vi "LABWAD.vi"() -> ()   [LabVIEW 2017]
uses:
  SubVIs/WAD_MainCluster.ctl
  SubVIs/TextureList.ctl
  SubVIs/PatchList.ctl
  SubVIs/Lumps.ctl
  Fire/Spread Fire.vi
  <vilib>/picture/picture.llb/Draw 8-Bit Pixmap.vi
  <userlib>/_OpenG.lib/array/array.llb/Filter 1D Array (String)__ogtk.vi
  <userlib>/_OpenG.lib/array/array.llb/Filter 1D Array with Scalar (String)__ogtk.vi
  <vilib>/regexp/Match Regular Expression.xnode
panel:
  out "2D Picture":picture
  in  "File Structure":string[](tree)
  out "Demonic Intensity Graph":i32[][](graph)
  # "Overview: Demonstrates how to read WAD files from original DOOM games.\nRequirements: LabVIEW Full Development System 2017 or compatible\nInstructions:\n1. Run this VI.\n2. Select a .wad file using the File > Open WAD File menu.\n3. Click on different items in the tree view to display them.\n4. Export the displayed image as PNG via drop-down menu on picture, or\n    select and export multiple items from the tree list via drop-down menu.\n5. Quit by using the File > Quit menu."
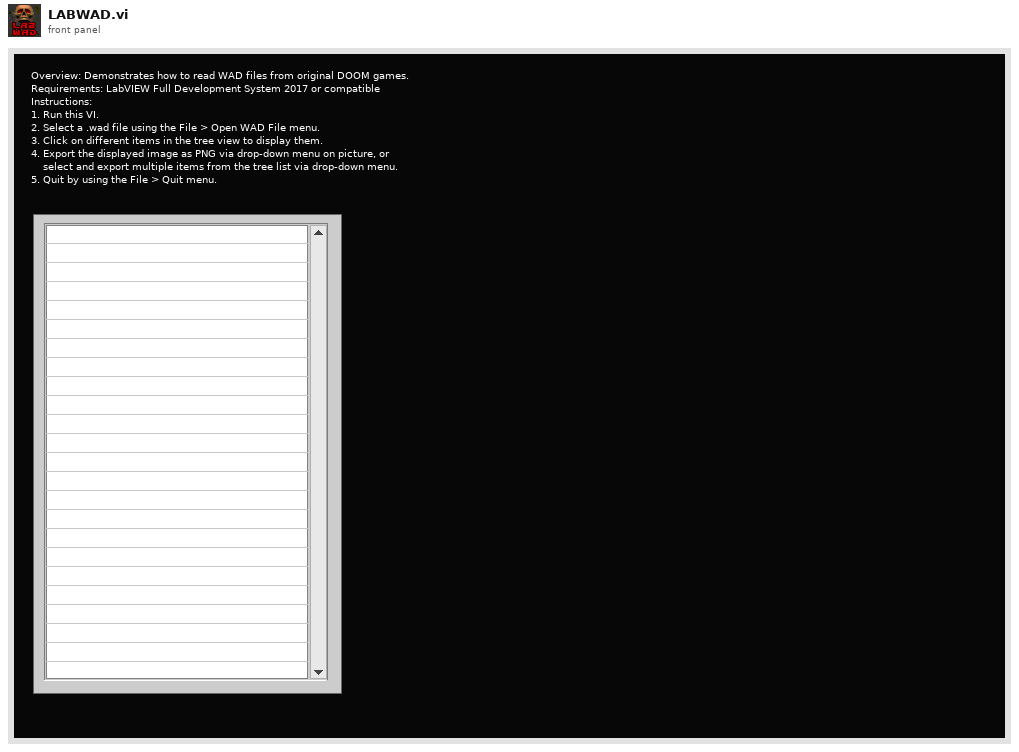
[diagram p1: front panel]
types:
  T1 = typedef "WAD_MainCluster.ctl" = cluster{"WAD file path":path, "WAD as U8 Array":u8[], "WAD Tree":refnum<vi>, "Palette":u32[], "TextureList":T2[], "PNAMES":string[], "Image Array":i16[][], "2D Picture":picture, "Lumps List":string[], "Lumps Array":T4[], "Textures Names":string[], "Image Mask":i16[][], "S_START Index":i32}
  T2 = typedef "TextureList.ctl" = cluster{"Name":string, "flags":u16, "masked":i16, "width":i16, "height":i16, "columndirectory":u32, "patchcount":i16, "PatchList":T3[]}
  T3 = typedef "PatchList.ctl" = cluster{"originx":i16, "originy":i16, "patch":i16}
  T4 = typedef "Lumps.ctl" = cluster{"offData":i32, "lenData":i32, "name":string}
  T5 = typedef "imagedata.ctl" = cluster{"image type":i32, "image depth":i32, "image":u8[], "mask":u8[], "colors":u32[], "Rectangle":cluster{"left":i16, "top":i16, "right":i16, "bottom":i16}}
  T6 = typedef "PatchHeader.ctl" = cluster{"Width":u16, "Height":u16, "XOffset":i16, "YOffset":i16}
  T7 = typedef "LVBoundsTypeDef.ctl" = cluster{"Width":u32, "Height":u32}
  T8 = cluster{"ItemTag":string, "Navigate Tree:Get Path":string[][]}
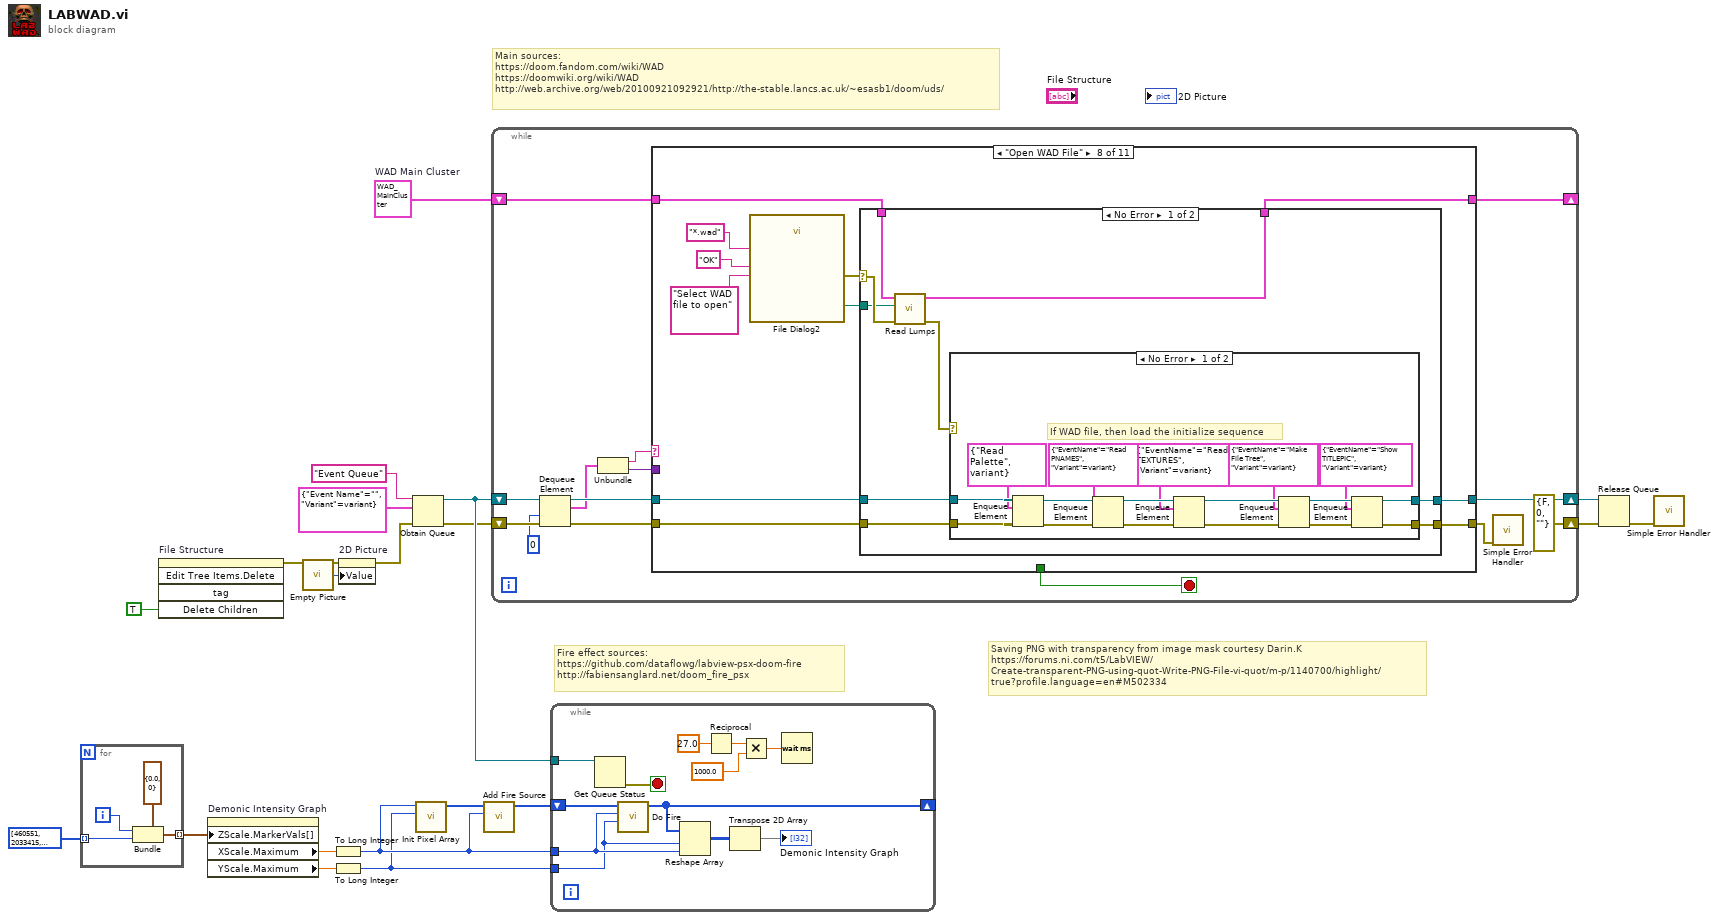
[diagram p0: block diagram]
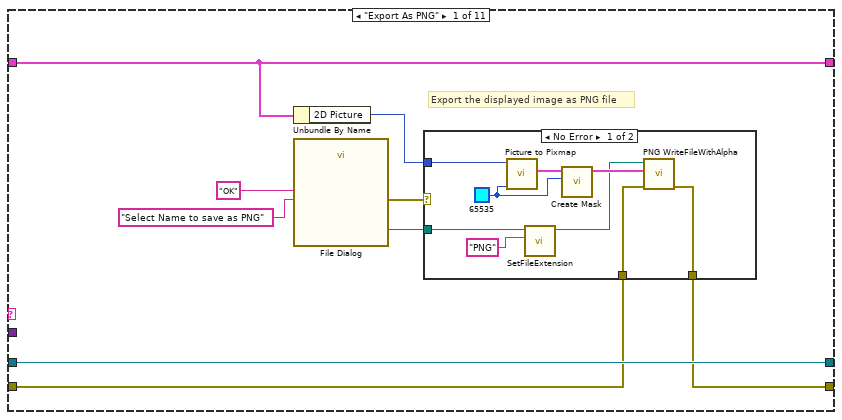
[diagram p2: hidden frame]
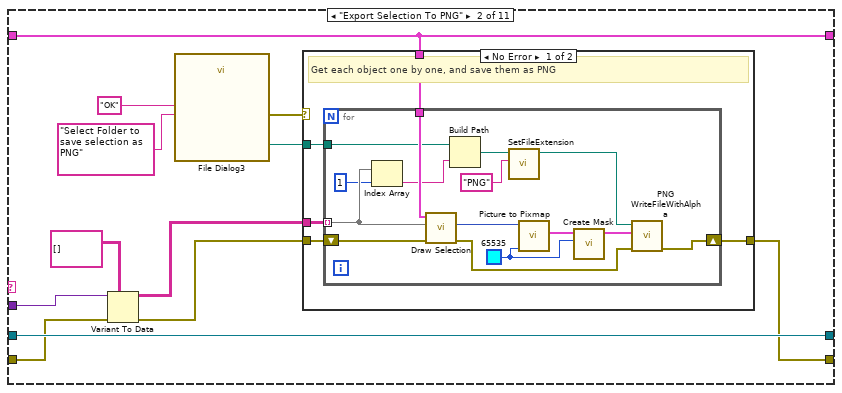
[diagram p4: hidden frame]
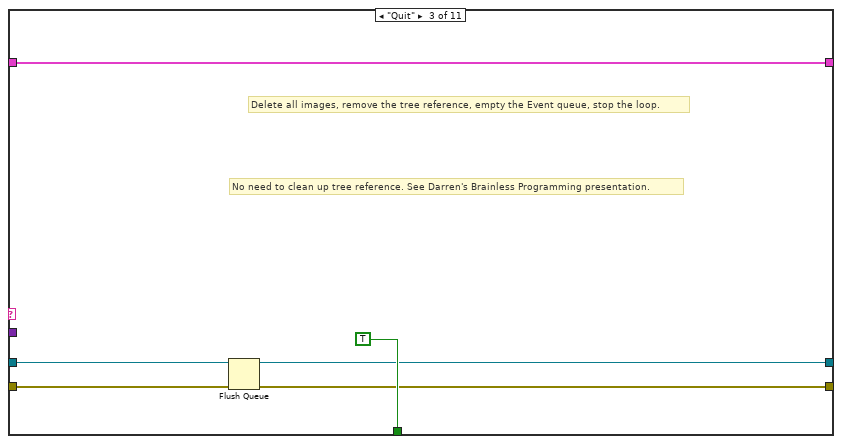
[diagram p6: hidden frame]
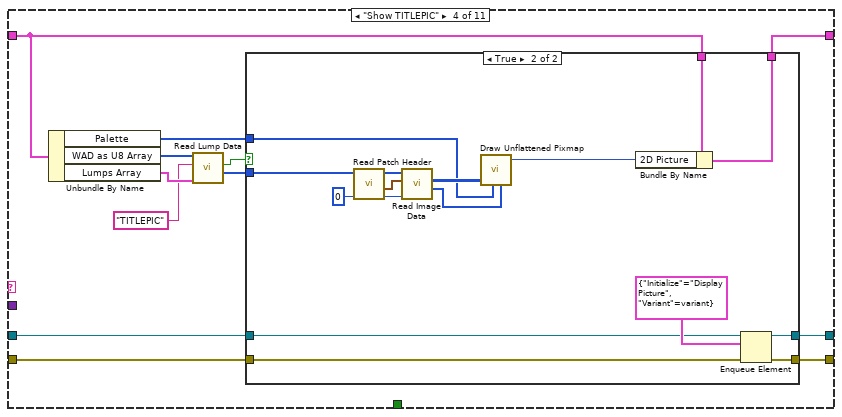
[diagram p7: hidden frame]
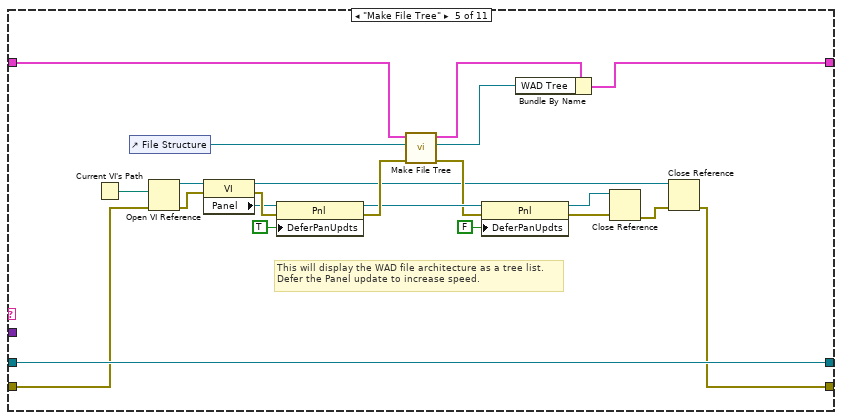
[diagram p9: hidden frame]
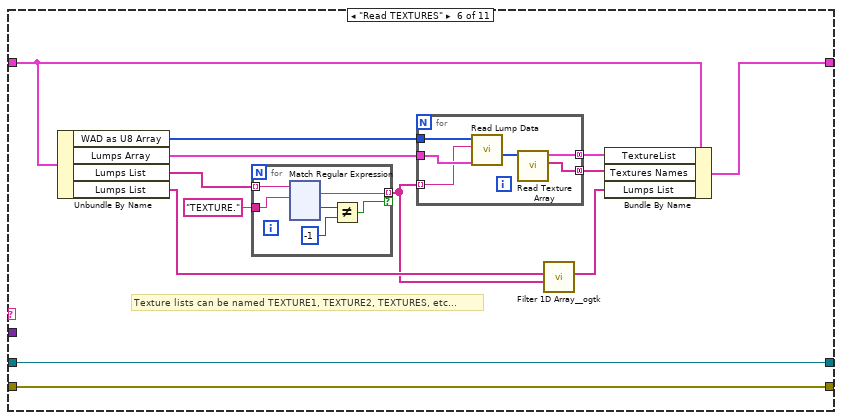
[diagram p10: hidden frame]
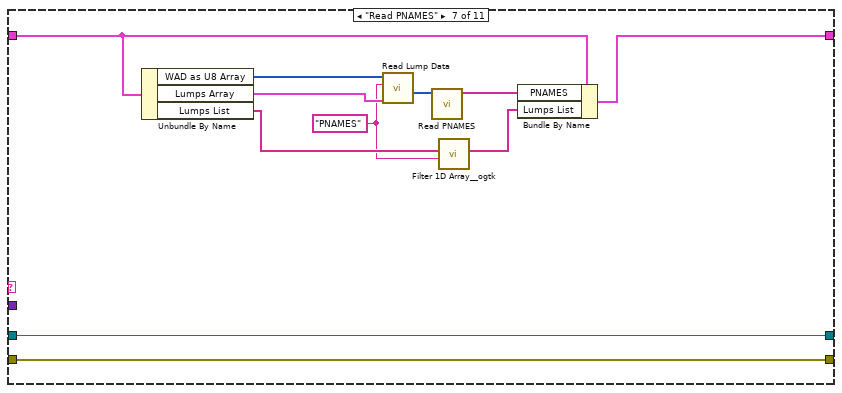
[diagram p11: hidden frame]
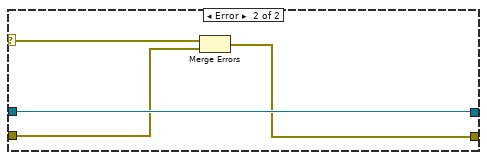
[diagram p12: hidden frame]
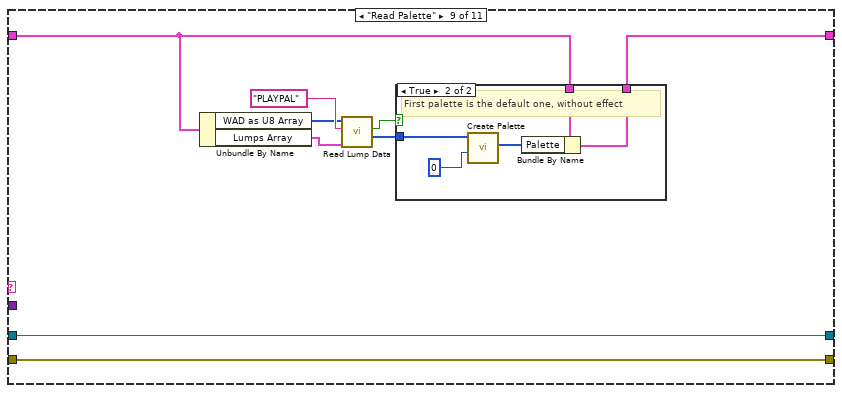
[diagram p14: hidden frame]
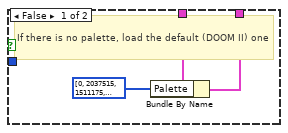
[diagram p15: hidden frame]
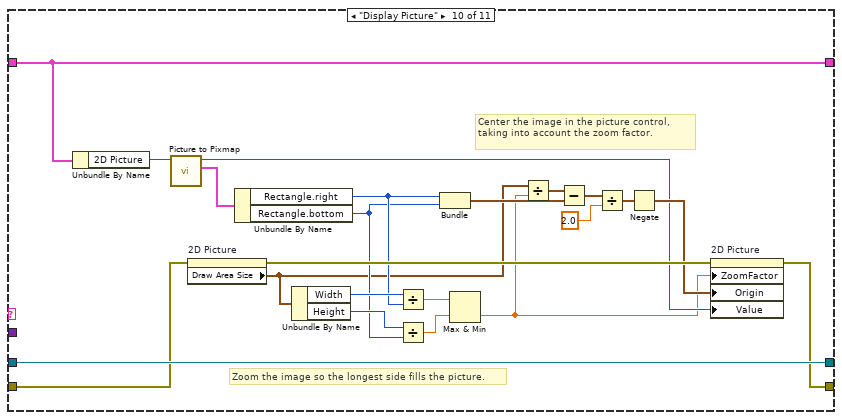
[diagram p16: hidden frame]
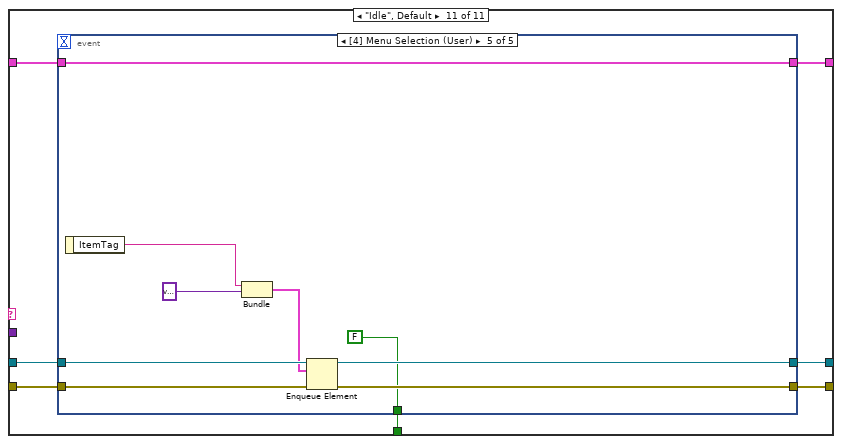
[diagram p17: hidden frame]
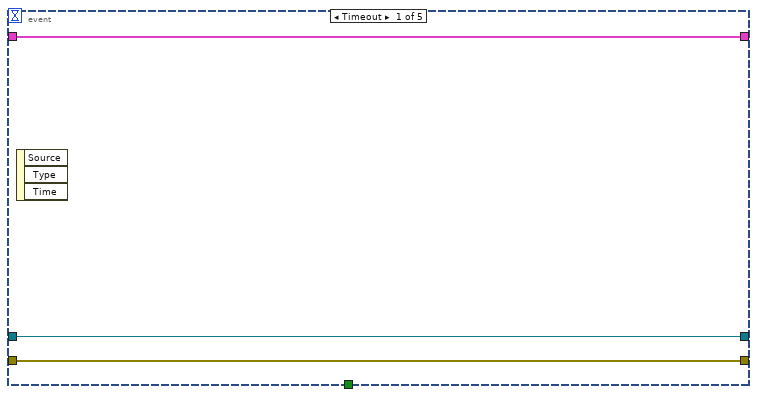
[diagram p18: hidden frame]
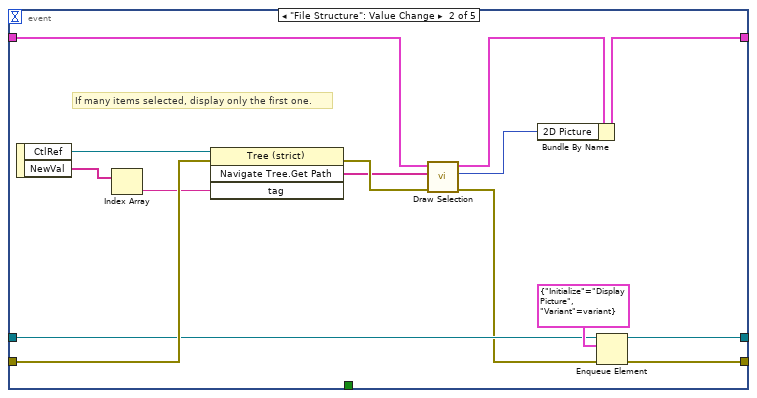
[diagram p19: hidden frame]
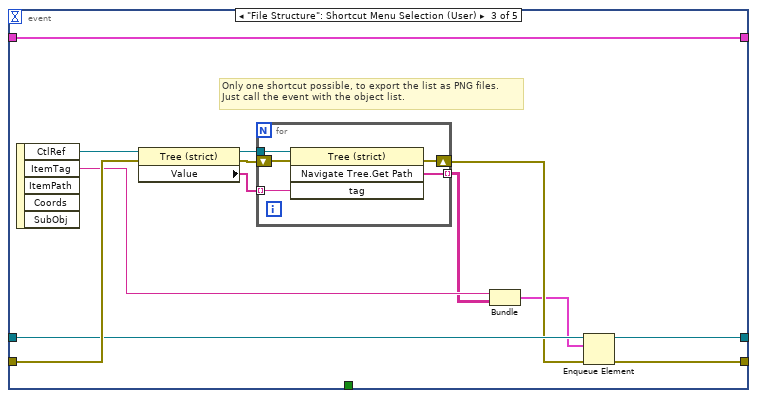
[diagram p20: hidden frame]
diagram:
  w19 = T1 {"WAD file path"=path "", "WAD as U8 Array"=[], "WAD Tree"=refnum, "Palette"=[], "TextureList"=[], "PNAMES"=[], "Image Array"=[], "2D Picture"=bytes[0], "Lumps List"=[], "Lumps Array"=[], "Textures Names"=[], "Image Mask"=[], "S_START Index"=0}  # WAD Main Cluster
  # "Fire effect sources:\nhttps://github.com/dataflowg/labview-psx-doom-fire\nhttp://fabiensanglard.net/doom_fire_psx"
  # "Saving PNG with transparency from image mask courtesy Darin.K\nhttps://forums.ni.com/t5/LabVIEW/Create-transparent-PNG-using-quot-Write-PNG-File-vi-quot/m-p/1140700/highlight/true?profile.language=en#M502334"
  # "Main sources:\nhttps://doom.fandom.com/wiki/WAD\nhttps://doomwiki.org/wiki/WAD\nhttp://web.archive.org/web/20100921092921/http://the-stable.lancs.ac.uk/~esasb1/doom/uds/"
  n1 = for {
    tunnel: u32[] [460551, 2033415, 3084039, 4656903, 5707527, 6758151, 7806727, 9381639, 10432263, 11484935, 12535559, 13059847, 14634759, 14636807, 14636807, 14114567, 14114567, 14116623, 13594383, 13596431, 13598479, 13600535, 13076247, 13078295, 13080351, 12558111, 12558111, 12560167, 12560167, 12562223, 12037935, 12039983, 12039991, 13619055, 14671775, 15724487, 16777215] ("Array") -> [w22] mode=indexing
    tunnel: [w21] -> w6 mode=indexing
    i -> [w23]
    n2 = Bundle(cluster=cluster{dbl, u32} {0.0, 0}, w23, w22) -> (w21:cluster{dbl, u32})
  }
  n3 = invoke on="File Structure" class="Tree (strict)" method="Edit Tree Items.Delete"("Delete Children"=TRUE ("Delete Children?")) -> (error out=w10:errorcluster)  [unwired: 4 in, 4 out]
  n4 = property on="Demonic Intensity Graph" class="IntGraph (strict)"("ZScale.MarkerVals[]"=w6) -> ("XScale.Maximum"=w8:dbl, "YScale.Maximum"=w7:dbl)  [unwired: 2 in, 2 out]
  n5 = call "Empty Picture"() -> ("empty picture"=w11:picture)
  n6 = To Long Integer(number=w8) -> (32bit integer=w5:i32)
  n7 = To Long Integer(number=w7) -> (32bit integer=w4:i32)
  n8 = property on="2D Picture" class="Pict"(error in=w10, "Value"=w11) -> (error out=w9:errorcluster)  [unwired: 1 in, 1 out]
  n9 = Obtain Queue(name (unnamed)="Event Queue", element data type=cluster{"Event Name":string, "Variant":variant} {"Event Name"="", "Variant"=variant}, error in (no error)=w9) -> (queue out=w14:refnum<queue>, error out=w13:errorcluster)  [unwired: 2 in, 1 out]
  n10 = call "Init Pixel Array.vi"("Height"=w4, "Width"=w5) -> ("Pixel Array"=w1:i32[])  [unwired: 9 in]
  n11 = call "Add Fire Source.vi"("Width"=w5, "Pixel Array In"=w1) -> ("Pixel Array Out"=w3:i32[])  [unwired: 9 in]
  n12 = while {
    shift-right: [w37] -> _
    shift-left: w19 -> [w38]
    shift-right: [w36] -> w16
    shift-left: w14 -> [w35]
    shift-right: [errorcluster {"status"=FALSE, "code"=0, "source"=""} ("error out")] -> w17
    shift-left: w13 -> [w34]
    stop <- w28 stop-if-true
    n13 = Dequeue Element(queue=w35, timeout in ms (-1)=0, error in (no error)=w34) -> (queue out=w32:refnum<queue>, element=w31:cluster{"Event Name":string, "Variant":variant}, error out=w33:errorcluster)  [unwired: 1 out]
    n14 = Unbundle(w31) -> ("Event Name"=w30:string, "Variant"=w29:variant)
    n15 = case shown="\"Open WAD File\"" w30 {
      tunnel: w38 -> [w46 w64 w96 w101 w148 w160 w294 w300 w346 w382 w389]
      tunnel: [w46 w64 w96 w100 w128 w159 w292 w310 w345 w382 w388] -> w37
      tunnel: w32 -> [w47 w69 w94 w108 w149 w162 w299 w306 w352 w381 w387]
      tunnel: [w47 w69 w92 w106 w149 w162 w299 w305 w352 w381 w386] -> w36
      tunnel: w33 -> [w39 w65 w93 w107 w140 w161 w298 w302 w351 w372 w385]
      tunnel: [w40 w60 w91 w105 w131 w161 w298 w304 w351 w380 w384] -> w25
      tunnel: w29 -> [_ w68 _ _ _ _ _ _ _ _ _]
      tunnel: [_ _ TRUE _ _ _ _ _ _ _ w383] -> w28
      frame "Export As PNG" {
        # "Export the displayed image as PNG file"
        n16 = Unbundle By Name(w46) -> ("2D Picture"=w45:picture)
        n17 = call "File Dialog"("prompt"="Select Name to save as PNG", "button label"="OK") -> ("selected path"=w42:path, "error out"=w41:errorcluster)  [unwired: 10 in, 2 out]
        n18 = case shown="No Error" w41 {
          tunnel: w45 -> [w51 _]
          tunnel: w42 -> [w56 _]
          tunnel: w39 -> [w49 w57]
          tunnel: [w48 w57] -> w40
          frame No Error {
            w52 = u32 65535 ("Background Color")
            n19 = call <vilib>:"Picture to Pixmap.vi"("Background Color"=w52, "picture"=w51) -> ("image data"=w54:T5)  [unwired: 8 in, 1 out]
            n20 = call "SetFileExtension.vi"("Extension"="PNG" ("button label"), "File path"=w56) -> ("FilePath with Extension"=w50:path)  [unwired: 9 in]
            n21 = call <vilib>:"Create Mask.vi"("Mask Color (Black)"=w52, "image data"=w54) -> ("image data"=w53:T5)  [unwired: 9 in]
            n22 = call "PNG WriteFileWithAlpha.vi"("error in (no error)"=w49, "image data"=w53, "Path to write (dialog)"=w50) -> ("error out"=w48:errorcluster)  [unwired: 7 in, 1 out]
          }
          frame Error {
          }
        }
      }
      frame "Export Selection To PNG" {
        n23 = Variant To Data(error in=w65, type=string[][] [] ("Navigate Tree:Get Path"), Variant=w68) -> (data=w66:string[][], error out=w58:errorcluster)
        n24 = call "File Dialog3"("prompt"="Select Folder to save selection as PNG", "button label"="OK") -> ("selected path"=w61:path, "error out"=w59:errorcluster)  [unwired: 10 in, 2 out]
        n25 = case shown="No Error" w59 {
          tunnel: w66 -> [w74 _]
          tunnel: w58 -> [w73 w90]
          tunnel: w64 -> [w72 _]
          tunnel: w61 -> [w71 _]
          tunnel: [w70 w90] -> w60
          frame No Error {
            # "Get each object one by one, and save them as PNG"
            n26 = for {
              tunnel: w74 -> [w85] mode=indexing
              shift-right: [w78] -> w70
              shift-left: w73 -> [w88]
              tunnel: w72 -> [w87]
              tunnel: w71 -> [w86]
              w75 = u32 65535 ("Background Color")
              n27 = Index Array(array=w85, index=1) -> (element=w83:string)
              n28 = call "Draw Selection.vi"("Error In"=w88, "Tree Path"=w85, "WAD Cluster IN"=w87) -> ("Error Out"=w79:errorcluster, "2D Picture"=w81:picture)  [unwired: 6 in, 1 out]
              n29 = Build Path(base path=w86, name or relative path=w83) -> (appended path=w82:path)
              n30 = call "SetFileExtension.vi"("Extension"="PNG" ("button label"), "File path"=w82) -> ("FilePath with Extension"=w80:path)  [unwired: 9 in]
              n31 = call <vilib>:"Picture to Pixmap.vi"("Background Color"=w75, "picture"=w81) -> ("image data"=w77:T5)  [unwired: 8 in, 1 out]
              n32 = call <vilib>:"Create Mask.vi"("Mask Color (Black)"=w75, "image data"=w77) -> ("image data"=w76:T5)  [unwired: 9 in]
              n33 = call "PNG WriteFileWithAlpha.vi"("error in (no error)"=w79, "image data"=w76, "Path to write (dialog)"=w80) -> ("error out"=w78:errorcluster)  [unwired: 7 in, 1 out]
            }
          }
          frame Error {
            # "If cancelled, don't do anything"
          }
        }
      }
      frame "Quit" {
        # "No need to clean up tree reference. See Darren's Brainless Programming presentation."
        # "Delete all images, remove the tree reference, empty the Event queue, stop the loop."
        n34 = Flush Queue(queue=w94, error in (no error)=w93) -> (queue out=w92:refnum<queue>, error out=w91:errorcluster)  [unwired: 1 out]
      }
      frame "Show TITLEPIC" {
        n35 = Unbundle By Name(w101) -> ("Palette"=w98:u32[], "WAD as U8 Array"=w104:u8[], "Lumps Array"=w103:T4[])
        n36 = call "Read Lump Data.vi"("Lumps Directory IN"=w103, "Lump Name"="TITLEPIC", "Input U8"=w104) -> ("Lump DATA OUT"=w102:u8[], "Found?"=w99:bool)  [unwired: 5 in, 2 out]
        n37 = case shown="True" w99 {
          tunnel: w108 -> [w110 w126]
          tunnel: w107 -> [w109 w113]
          tunnel: [w110 w125] -> w106
          tunnel: [w109 w124] -> w105
          tunnel: w102 -> [_ w123]
          tunnel: w101 -> [w111 w118]
          tunnel: [w111 w117] -> w100
          tunnel: w98 -> [_ w115]
          frame False {
          }
          frame True {
            n38 = call "Read Patch Header.vi"("Index"=u32 0, "Patch DATA IN"=w123) -> ("Index+8"=w119:u32, "PatchHeader"=w122:T6, "Patch DATA OUT"=w121:u8[])  [unwired: 7 in]
            n39 = call "Read Image Data.vi"("Input Index"=w119, "PatchHeader"=w122, "Patch DATA IN"=w121) -> ("Mask OUT"=w114:u8[], "Image OUT"=w116:u8[][])  [unwired: 5 in, 2 out]
            n40 = call-poly <vilib>:"Draw Unflattened Pixmap.vi"("data"=w116, "color table"=w115, "mask"=w114) -> ("new picture"=w112:picture)  [unwired: 6 in]
            n41 = Bundle By Name(cluster=w118, "2D Picture"=w112) -> (w117:T1)
            n42 = Enqueue Element(queue=w126, element=cluster{"Initialize":string, "Variant":variant} {"Initialize"="Display Picture", "Variant"=variant}, error in (no error)=w113) -> (queue out=w125:refnum<queue>, error out=w124:errorcluster)  [unwired: 1 in, 1 out]
          }
        }
      }
      frame "Make File Tree" {
        # "This will display the WAD file architecture as a tree list.\nDefer the Panel update to increase speed."
        n43 = Current VI's Path() -> (path=w142:path)
        n44 = control-ref of="File Structure"() -> (w147:refnum<vi>)
        n45 = Open VI Reference(vi path=w142, error in (no error)=w140) -> (vi reference=w143:refnum<vi>, error out=w145:errorcluster)  [unwired: 4 in]
        n46 = property class="VI"(reference=w143, error in=w145) -> (reference out=w132:refnum<vi>, error out=w146:errorcluster, "Panel"=w144:refnum<vi>)
        n47 = property class="Pnl"(reference=w144, error in=w146, "DeferPanUpdts"=TRUE ("Defer Panel Updates")) -> (reference out=w137:refnum<vi>, error out=w139:errorcluster)
        n48 = call "Make File Tree.vi"("Error In"=w139, "TreeControl in"=w147, "WAD Main Cluster"=w148) -> ("Error Out"=w136:errorcluster, "TreeControl OUT"=w129:refnum<vi>, "WAD Main Cluster OUT"=w130:T1)  [unwired: 6 in]
        n49 = property class="Pnl"(reference=w137, error in=w136, "DeferPanUpdts"=FALSE ("Defer Panel Updates")) -> (reference out=w134:refnum<vi>, error out=w135:errorcluster)
        n50 = Bundle By Name(cluster=w130, "WAD Tree"=w129) -> (w128:T1)
        n51 = Close Reference(reference=w134, error in (no error)=w135) -> (error out=w133:errorcluster)
        n52 = Close Reference(reference=w132, error in (no error)=w133) -> (error out=w131:errorcluster)
      }
      frame "Read TEXTURES" {
        # "Texture lists can be named TEXTURE1, TEXTURE2, TEXTURES, etc..."
        n53 = Unbundle By Name(w160) -> ("WAD as U8 Array"=w158:u8[], "Lumps Array"=w157:T4[], "Lumps List"=w155:string[], "Lumps List"=w152:string[])
        n54 = for {
          tunnel: w155 -> [w173] mode=indexing
          tunnel: "TEXTURE." ("format string") -> [w174]
          tunnel: [w172] -> w151 mode=indexing if=w169
          n55 = xnode "Match Regular Expression"("input string"=w173, "regular expression"=w174) -> ("whole match"=w172:string, "offset past match"=w171:i32)  [unwired: 4 in, 3 out]
          n56 = Not Equal?(x=w171, y=-1) -> (x != y?=w169:bool)
        }
        n57 = for {
          tunnel: w158 -> [w167]
          tunnel: w157 -> [w166]
          tunnel: [w165] -> w154 mode=concatenating
          tunnel: [w164] -> w153 mode=concatenating
          tunnel: w151 -> [w163] mode=indexing
          n58 = call "Read Lump Data.vi"("Lumps Directory IN"=w166, "Lump Name"=w163, "Input U8"=w167) -> ("Lump DATA OUT"=w168:u8[])  [unwired: 5 in, 3 out]
          n59 = call "Read Texture Array.vi"("TEXTURES Lump"=w168) -> ("Texture Names Array"=w164:string[], "Textures array"=w165:T2[])  [unwired: 9 in]
        }
        n60 = call-poly <userlib>:"Filter 1D Array__ogtk.vi"("items to filter"=w151, "array"=w152) -> ("filtered array"=w150:string[])  [unwired: 4 in, 1 out]
        n61 = Bundle By Name(cluster=w160, "TextureList"=w154, "Textures Names"=w153, "Lumps List"=w150) -> (w159:T1)
      }
      frame "Read PNAMES" {
        w290 = "PNAMES" ("element")
        n62 = Unbundle By Name(w294) -> ("WAD as U8 Array"=w296:u8[], "Lumps Array"=w295:T4[], "Lumps List"=w291:string[])
        n63 = call "Read Lump Data.vi"("Lumps Directory IN"=w295, "Lump Name"=w290, "Input U8"=w296) -> ("Lump DATA OUT"=w297:u8[])  [unwired: 5 in, 3 out]
        n64 = call "Read PNAMES.vi"("Lump DATA IN"=w297) -> ("PNAMES Array"=w293:string[])  [unwired: 10 in]
        n65 = call-poly <userlib>:"Filter 1D Array__ogtk.vi"("items to filter"=w290, "array"=w291) -> ("filtered array"=w289:string[])  [unwired: 4 in, 1 out]
        n66 = Bundle By Name(cluster=w294, "PNAMES"=w293, "Lumps List"=w289) -> (w292:T1)
      }
      frame "Open WAD File" {
        n67 = call "File Dialog2"("prompt"="Select WAD file to open", "button label"="OK", "pattern (all files)"="*.wad") -> ("selected path"=w308:path, "error out"=w303:errorcluster)  [unwired: 9 in, 2 out]
        n68 = case shown="No Error" w303 {
          selector: w303 -> [w314 _]
          tunnel: [w311 w342] -> w310
          tunnel: w308 -> [w313 _]
          tunnel: w306 -> [w319 w343]
          tunnel: w302 -> [w318 w341]
          tunnel: [w317 w343] -> w305
          tunnel: [w316 w341] -> w304
          tunnel: w300 -> [w312 w342]
          frame No Error {
            n69 = call "Read Lumps.vi"("Error In"=w314, "file (use dialog)"=w313, "Cluster"=w312) -> ("Error Out"=w315:errorcluster, "Cluster 2"=w311:T1)  [unwired: 7 in]
            n70 = case shown="No Error" w315 {
              selector: w315 -> [_ w339]
              tunnel: w319 -> [w323 w340]
              tunnel: w318 -> [w322 w338]
              tunnel: [w321 w340] -> w317
              tunnel: [w320 w337] -> w316
              frame No Error {
                # "If WAD file, then load the initialize sequence"
                n71 = Enqueue Element(queue=w323, element=cluster{"EventName":string, "Variant":variant} {"EventName"="Read Palette", "Variant"=variant}, error in (no error)=w322) -> (queue out=w334:refnum<queue>, error out=w333:errorcluster)  [unwired: 1 in, 1 out]
                n72 = Enqueue Element(queue=w334, element=cluster{"EventName":string, "Variant":variant} {"EventName"="Read PNAMES", "Variant"=variant}, error in (no error)=w333) -> (queue out=w336:refnum<queue>, error out=w335:errorcluster)  [unwired: 1 in, 1 out]
                n73 = Enqueue Element(queue=w336, element=cluster{"EventName":string, "Variant":variant} {"EventName"="Read TEXTURES", "Variant"=variant}, error in (no error)=w335) -> (queue out=w330:refnum<queue>, error out=w329:errorcluster)  [unwired: 1 in, 1 out]
                n74 = Enqueue Element(queue=w330, element=cluster{"EventName":string, "Variant":variant} {"EventName"="Make File Tree", "Variant"=variant}, error in (no error)=w329) -> (queue out=w332:refnum<queue>, error out=w331:errorcluster)  [unwired: 1 in, 1 out]
                n75 = Enqueue Element(queue=w332, element=cluster{"EventName":string, "Variant":variant} {"EventName"="Show TITLEPIC", "Variant"=variant}, error in (no error)=w331) -> (queue out=w321:refnum<queue>, error out=w320:errorcluster)  [unwired: 1 in, 1 out]
              }
              frame Error {
                n76 = Merge Errors(w339, w338) -> (w337:errorcluster)
              }
            }
          }
          frame Error {
          }
        }
      }
      frame "Read Palette" {
        n77 = Unbundle By Name(w346) -> ("WAD as U8 Array"=w349:u8[], "Lumps Array"=w348:T4[])
        n78 = call "Read Lump Data.vi"("Lumps Directory IN"=w348, "Lump Name"="PLAYPAL" ("element"), "Input U8"=w349) -> ("Lump DATA OUT"=w347:u8[], "Found?"=w344:bool)  [unwired: 5 in, 2 out]
        n79 = case shown="True" w344 {
          tunnel: w347 -> [_ w359]
          tunnel: w346 -> [w355 w358]
          tunnel: [w354 w356] -> w345
          frame False {
            # "If there is no palette, load the default (DOOM II) one"
            n80 = Bundle By Name(cluster=w355, "Palette"=u32[] [0, 2037515, 1511175, 4934475, 16777215, 1776411, 1250067, 723723, 460551, 3094303, 2304783, 1515271, 988928, 5192491, 4666147, 4139803, 16758711, 16231339, 15967139, 15439767, 15175567, 14649223, 14383995, 13857651, 13331307, 13067107, 12540763, 12277591, 11751247, 11487047, 10960703, 10697531, 10171187, 9908015, 9382699, 9118499, 8593183, 8330011, 7804695, 7541523, 7016207, 6753035, 6227719, 5965575, 5441287, 5177344, 4653056, 4390912, 16772063, 16770003, 16767943, 16765883, 16764851, 16762791, 16760731, 16759699, 16757635, 16231291, 15704947, 15178603, 14652259, 14125915, 13599571, 13336399, 12548939, 11760455, 11235139, 10709823, 10183483, 9396023, 8869683, 8344367, 7819051, 7030567, 6243107, 5455647, 4929307, 4140823, 3353363, 2827023, 15724527, 15198183, 14671839, 14408667, 13882323, 13355979, 13092807, 12566463, 12040119, 11776947, 11250603, 10987431, 10461087, 9934743, 9671571, 9145227, 8618883, 8355711, 7829367, 7303023, 7039851, 6513507, 5987163, 5723991, 5197647, 4671303, 4408131, 3881787, 3618615, 3092271, 2565927, 2302755, 7864175, 7335783, 6807391, 6278999, 6012751, 5484359, 4955967, 4428599, 4162351, 3633963, 3105571, 2577179, 2048791, 1520399, 1254155, 726791, 12560271, 12033927, 11507583, 10981239, 10454895, 10190699, 9665379, 9139035, 8612695, 8086351, 7823179, 7296835, 6771519, 6245175, 5718835, 5455663, 10453859, 9402195, 8612683, 7823167, 6771507, 5981995, 5192483, 4403995, 8093539, 7304023, 6777679, 5989191, 5461819, 4673331, 4146987, 3620647, 16777075, 15457111, 14138179, 12819247, 11500319, 10181395, 8864519, 7547648, 16777215, 16767963, 16759739, 16751515, 16743291, 16736095, 16727871, 16719647, 16711680, 15663104, 14876672, 14090240, 13303808, 12517376, 11730944, 10944512, 10158080, 9109504, 8323072, 7536640, 6750208, 5963776, 5177344, 4390912, 15198207, 13092863, 11250687, 9408511, 7566335, 5460991, 3618815, 1776639, 255, 227, 203, 179, 155, 131, 107, 83, 16777215, 16772059, 16766907, 16762779, 16757627, 16753499, 16748347, 16744219, 15954711, 15429391, 14640911, 14114571, 13326087, 12799744, 12011264, 11485952, 16777215, 16777175, 16777139, 16777103, 16777067, 16777031, 16776995, 16776960, 10960640, 10434304, 9645824, 8856320, 5192487, 4402971, 3613459, 3087115, 83, 71, 59, 47, 35, 23, 11, 0, 16752451, 16770891, 16743423, 16711935, 13566159, 10420379, 7274603, 10972011] ("Doom 2 Palette")) -> (w354:T1)
          }
          frame True {
            # "First palette is the default one, without effect"
            n81 = call "Create Palette.vi"("Palette Index"=0 ("index"), "Palette Lump"=w359) -> ("Palette"=w357:u32[])  [unwired: 9 in]
            n82 = Bundle By Name(cluster=w358, "Palette"=w357) -> (w356:T1)
          }
        }
      }
      frame "Display Picture" {
        # "Center the image in the picture control, taking into account the zoom factor."
        # "Zoom the image so the longest side fills the picture."
        n83 = Unbundle By Name(w382) -> ("2D Picture"=w379:picture)
        n84 = call <vilib>:"Picture to Pixmap.vi"("picture"=w379) -> ("image data"=w378:T5, "new picture"=w363:picture)  [unwired: 9 in]
        n85 = property on="2D Picture" class="Pict"(error in=w372) -> (error out=w373:errorcluster, "Draw Area Size"=w361:T7)  [unwired: 1 in, 1 out]
        n86 = Unbundle By Name(w378) -> ("Rectangle.right"=w370:i16, "Rectangle.bottom"=w369:i16)
        n87 = Unbundle By Name(w361) -> ("Width"=w377:u32, "Height"=w376:u32)
        n88 = Divide(x=w377, y=w370) -> (x/y=w375:dbl)
        n89 = Divide(x=w376, y=w369) -> (x/y=w374:dbl)
        n90 = Bundle("right"=w370, "bottom"=w369) -> (w368:cluster{"right":i16, "bottom":i16})  [unwired: 1 in]
        n91 = Max & Min(x=w375, y=w374) -> (min(x,y)=w362:dbl)  [unwired: 1 out]
        n92 = Divide(x=w361, y=w362) -> (x/y=w371:cluster{"Width":dbl, "Height":dbl})
        n93 = Subtract(x=w371, y=w368) -> (x-y=w367:cluster{dbl, dbl})
        n94 = Divide(x=w367, y=2.0) -> (x/y=w365:cluster{dbl, dbl})
        n95 = Negate(x=w365) -> (-x=w364:cluster{dbl, dbl})
        n96 = property on="2D Picture" class="Pict"(error in=w373, "ZoomFactor"=w362, "Origin"=w364, "Value"=w363) -> (error out=w380:errorcluster)  [unwired: 1 in, 1 out]
      }
      frame "Idle", Default {
        n97 = event shown="[4] Menu Selection (User)" {
          selector: _ -> [_ _ _ _ _]
          dyn-events: _ -> [_ _ _ _ _]
          timeout: _ -> [_ _ _ _ _]
          tunnel: w389 -> [w392 w405 w415 w433 w442]
          tunnel: [w392 w399 w415 w433 w442] -> w388
          tunnel: w387 -> [w391 w397 w414 w432 w441]
          tunnel: [w391 w396 w412 w430 w439] -> w386
          tunnel: w385 -> [w390 w403 w419 w431 w440]
          tunnel: [w390 w394 w411 w429 w438] -> w384
          tunnel: [_ _ _ _ FALSE] -> w383
          event Timeout {
            n98 = event-data() -> ()  [unwired: 1 in, 3 out]
          }
          event "File Structure": Value Change {
            # "If many items selected, display only the first one."
            n99 = event-data() -> ("CtlRef"=w404:refnum<vi>, "NewVal"=w402:string[])  [unwired: 1 in]
            n100 = Index Array(array=w402) -> (element=w401:string)  [unwired: 1 in]
            n101 = invoke class="Tree (strict)" method="Navigate Tree.Get Path"(reference=w404, error in=w403, "tag"=w401) -> (error out=w407:errorcluster, "Navigate Tree:Get Path"=w406:string[])  [unwired: 1 in, 2 out]
            n102 = call "Draw Selection.vi"("Error In"=w407, "Tree Path"=w406, "WAD Cluster IN"=w405) -> ("Error Out"=w395:errorcluster, "2D Picture"=w393:picture, "WAD Cluster OUT"=w400:T1)  [unwired: 6 in]
            n103 = Bundle By Name(cluster=w400, "2D Picture"=w393) -> (w399:T1)
            n104 = Enqueue Element(queue=w397, element=cluster{"Initialize":string, "Variant":variant} {"Initialize"="Display Picture", "Variant"=variant}, error in (no error)=w395) -> (queue out=w396:refnum<queue>, error out=w394:errorcluster)  [unwired: 1 in, 1 out]
          }
          event "File Structure": Shortcut Menu Selection (User) {
            # "Only one shortcut possible, to export the list as PNG files.\nJust call the event with the object list."
            n105 = event-data() -> ("CtlRef"=w420:refnum<vi>, "ItemTag"=w410:string)  [unwired: 1 in, 3 out]
            n106 = property class="Tree (strict)"(reference=w420, error in=w419) -> (reference out=w418:refnum<vi>, error out=w417:errorcluster, "Value"=w416:string[])
            n107 = for {
              tunnel: w418 -> [w425]
              tunnel: w416 -> [w423] mode=indexing
              shift-right: [w422] -> w413
              shift-left: w417 -> [w424]
              tunnel: [w421] -> w409 mode=indexing
              n108 = invoke class="Tree (strict)" method="Navigate Tree.Get Path"(reference=w425, error in=w424, "tag"=w423) -> (error out=w422:errorcluster, "Navigate Tree:Get Path"=w421:string[])  [unwired: 1 in, 2 out]
            }
            n109 = Bundle("ItemTag"=w410, "Navigate Tree:Get Path"=w409) -> (w408:T8)  [unwired: 1 in]
            n110 = Enqueue Element(queue=w414, element=w408, error in (no error)=w413) -> (queue out=w412:refnum<queue>, error out=w411:errorcluster)  [unwired: 1 in, 1 out]
          }
          event "2D Picture": Shortcut Menu Selection (User) {
            # "Only one shortcut: export as PNG"
            n111 = event-data() -> ("ItemTag"=w428:string)  [unwired: 1 in]
            n112 = Bundle("ItemTag"=w428, "Variant"=variant) -> (w426:cluster{"ItemTag":string, "Variant":variant})  [unwired: 1 in]
            n113 = Enqueue Element(queue=w432, element=w426, error in (no error)=w431) -> (queue out=w430:refnum<queue>, error out=w429:errorcluster)  [unwired: 1 in, 1 out]
          }
          event Menu Selection (User) {
            n114 = event-data() -> ("ItemTag"=w437:string)  [unwired: 1 in]
            n115 = Bundle("ItemTag"=w437, "Variant"=variant) -> (w435:cluster{"ItemTag":string, "Variant":variant})  [unwired: 1 in]
            n116 = Enqueue Element(queue=w441, element=w435, error in (no error)=w440) -> (queue out=w439:refnum<queue>, error out=w438:errorcluster)  [unwired: 1 in, 1 out]
          }
        }
      }
    }
    n117 = call <vilib>:"Simple Error Handler.vi"("error in (no error)"=w25) -> ()  [unwired: 4 in, 5 out]
  }
  n118 = while {
    shift-right: [w449] -> _
    shift-left: w3 -> [w443]
    tunnel: w5 -> [w448]
    tunnel: w4 -> [w447]
    tunnel: w14 -> [w446]
    stop <- w445 stop-if-true
    n119 = Get Queue Status(queue=w446) -> (error out=w445:errorcluster)  [unwired: 2 in, 7 out]
    n120 = call "Do Fire.vi"("Height"=w447, "Width"=w448, "Pixel Array In"=w443) -> ("Pixel Array Out"=w449:i32[])  [unwired: 8 in]
    n121 = Reshape Array(w449, w447, w448) -> (w451:i32[][])
    n122 = Reciprocal(x=27.0) -> (1/x=w454:dbl)
    n123 = Transpose 2D Array(2D array=w451) -> (transposed array=→"Demonic Intensity Graph":i32[][])
    n124 = Multiply(x=w454, y=1000.0) -> (x*y=w452:dbl)
    n125 = Wait (ms)(milliseconds to wait=w452) -> ()  [unwired: 1 out]
  }
  n126 = Release Queue(queue=w16, error in (no error)=w17) -> (error out=w15:errorcluster)  [unwired: 1 in, 2 out]
  n127 = call <vilib>:"Simple Error Handler.vi"("error in (no error)"=w15) -> ()  [unwired: 4 in, 5 out]
